vi "OutputChromaError.vi"(7 "PluginID":string, 8 "error in (no error)":errorcluster, 10 "Chroma Output String":string, 11 "Initial Message String":string) -> (0 "error out":errorcluster, 3 "Output String":string)   [LabVIEW 2018, in "AcPwrModule.lvlib"]
uses:
  AcPwrModule.lvlib
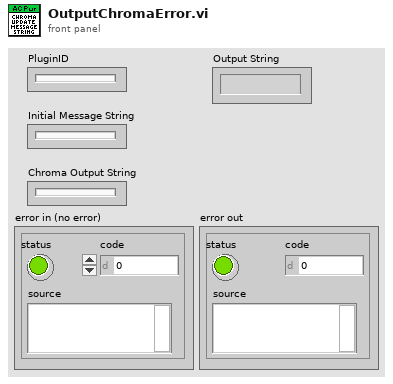
[diagram p1: front panel]
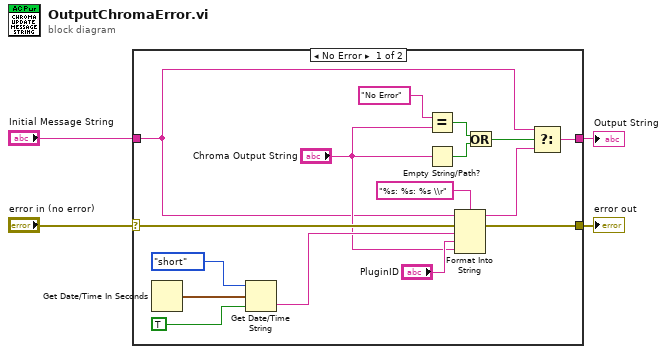
[diagram p0: block diagram]
diagram:
  n1 = case shown="No Error" "error in (no error)" {
    selector: "error in (no error)" -> [w11 w22]
    tunnel: [w20 w22] -> w4
    tunnel: "Initial Message String" -> [w5 w21]
    tunnel: [w6 w21] -> w1
    frame No Error {
      n2 = Get Date/Time In Seconds() -> (seconds since 1Jan1904=w13:timestamp)
      n3 = Get Date/Time String(date format (0)=enum16{"short", "long", "abbreviated"}."short", seconds (now)=w13, want seconds? (F)=TRUE) -> (time string=w15:string)  [unwired: 1 out]
      n4 = Equal?(x="No Error", y="Chroma Output String") -> (x = y?=w17:bool)
      n5 = Empty String/Path?(string/path="Chroma Output String") -> (empty?=w18:bool)
      n6 = Format Into String(format string="%s: %s: %s \\r", initial string=w5, error in=w11, w15, "PluginID", "Chroma Output String") -> (resulting string=w7:string, error out=w20:errorcluster)
      n7 = Or(x=w17, y=w18) -> (x .or. y?=w19:bool)
      n8 = Select(t=w5, s=w19, f=w7) -> (s? t:f=w6:string)
    }
    frame Error {
    }
  }
  "error out" <- w4
  "Output String" <- w1
